vi "doAction.vi"(8 "error in (no error)":errorcluster, 10 "ContextData":refnum<class "ContextData.lvclass">, 11 "Run in":refnum<class "Check Move.lvclass">) -> (0 "error out":errorcluster, 2 "ContextData Out":refnum<class "ContextData.lvclass">, 3 "Run out":refnum<class "Check Move.lvclass">)   [LabVIEW 2019, in "Check Move.lvclass"]
uses:
  Check Move.lvclass
  ContextData/ContextData.lvclass
  Check Move.lvclass/Check Move.ctl
  Simon_Engine/Simon_Engine.lvclass
  Messages/simonMessages/simonMessages.lvclass
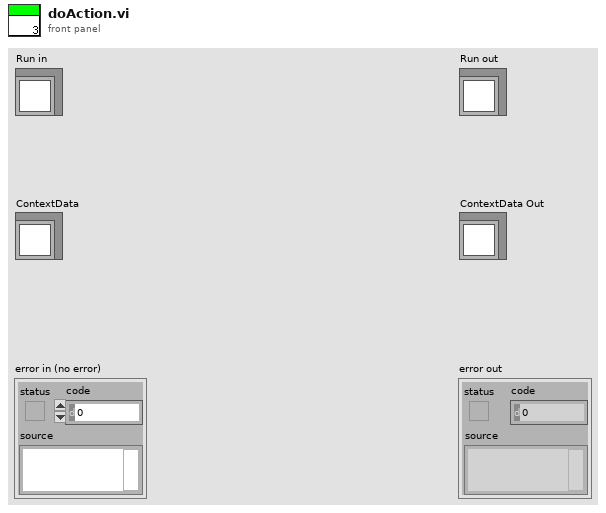
[diagram p1: front panel]
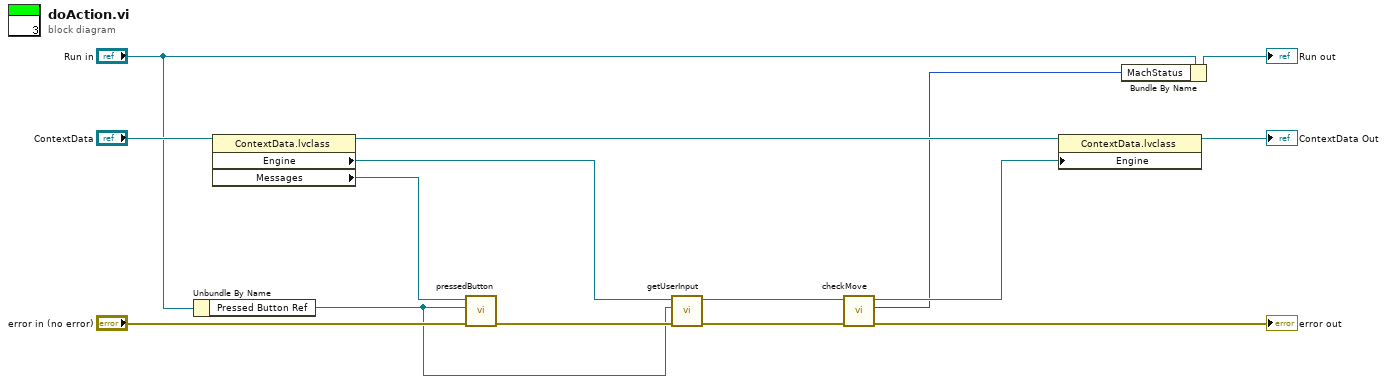
[diagram p0: block diagram]
diagram:
  n1 = Unbundle By Name("Run in") -> ("Pressed Button Ref"=w1:refnum<vi>)
  n2 = property class="ContextData.lvclass"(reference="ContextData") -> (reference out=w14:refnum<class "ContextData.lvclass">, "Engine"=w6:refnum<class "Simon_Engine.lvclass">, "Messages"=w3:refnum<class "simonMessages.lvclass">)  [unwired: 1 in, 1 out]
  n3 = call "pressedButton.vi"("error in (no error)"="error in (no error)", "Bool Refnum"=w1, "simonMessages in"=w3) -> ("error out"=w4:errorcluster)  [unwired: 7 in, 1 out]
  n4 = call-dynamic "getUserInput.vi"("error in (no error)"=w4, "clickedLEDReference"=w1, "Simon_Engine in"=w6) -> ("error out"=w7:errorcluster, "Simon_Engine out"=w5:refnum<class "Simon_Engine.lvclass">)  [unwired: 7 in]
  n5 = call-dynamic "checkMove.vi"("error in (no error)"=w7, "Simon_Engine in"=w5) -> ("error out"=→"error out":errorcluster, "MachStatus"=w10:i16, "Simon_Engine out"=w11:refnum<class "Simon_Engine.lvclass">)  [unwired: 7 in]
  n6 = property class="ContextData.lvclass"(reference=w14, "Engine"=w11) -> (reference out=→"ContextData Out":refnum<class "ContextData.lvclass">)  [unwired: 1 in, 1 out]
  n7 = Bundle By Name(cluster="Run in", "MachStatus"=w10) -> (→"Run out":refnum<class "Check Move.lvclass">)
